vi "stitchingModeSimple_KJM.vi"(9 "Data In":dbl[][][](array[numeric])) -> (2 "Stitched Data Out":dbl[][](array[numeric]))   [LabVIEW 2020]
doc: "Stitches spectra based on simple cut-off modus."
uses:
  CCD.lvclass/CCD.ctl
  4c98e68f-fed8-44bd-a6f6-c5aabdf5d44d.vi
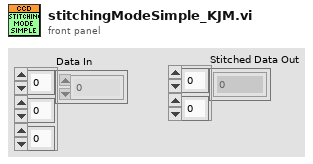
[diagram p1: front panel]
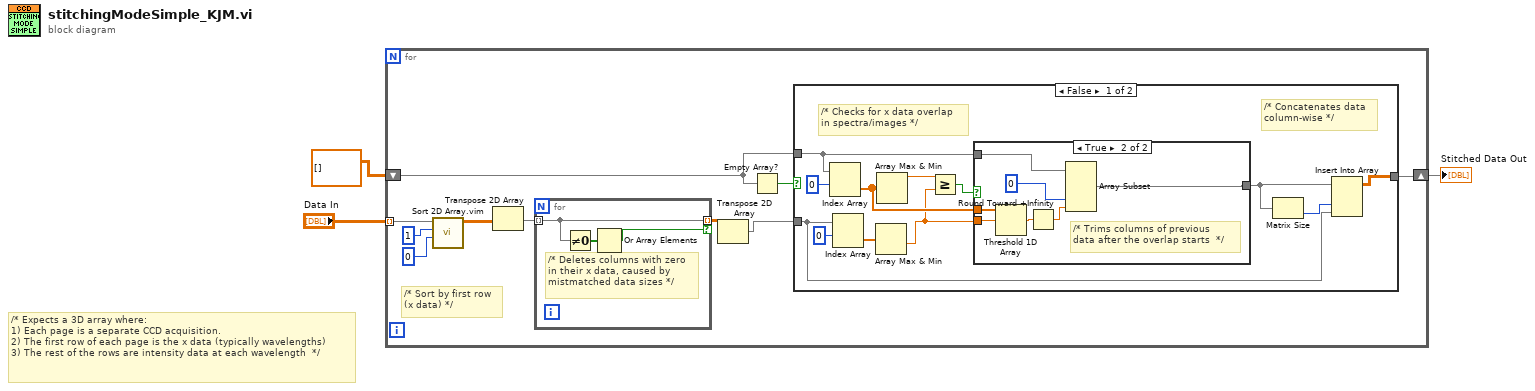
[diagram p0: block diagram]
diagram:
  # "/* Expects a 3D array where:\n1) Each page is a separate CCD acquisition.\n2) The first row of each page is the x data (typically wavelengths)\n3) The rest of the rows are intensity data at each wavelength  */"
  n1 = for {
    tunnel: "Data In" -> [w6] mode=indexing
    shift-right: [w13] -> w2
    shift-left: dbl[][] [] ("Empty Array") -> [w11]
    # "/* Sort by first row \n(x data) */"
    n2 = call "Sort 2D Array.vim"("index"=0, "dimension to index (column)"=1 ("index"), "2D array"=w6) -> ("sorted 2D array"=w5:dbl[][])  [unwired: 7 in, 1 out]
    n3 = Transpose 2D Array(2D array=w5) -> (transposed array=w10:dbl[][])
    n4 = for {
      tunnel: w10 -> [w15] mode=indexing
      tunnel: [w15] -> w9 mode=indexing if=w16
      # "/* Deletes columns with zero\nin their x data, caused by\nmistmatched data sizes */"
      n5 = Not Equal To 0?(x=w15) -> (x != 0?=w14:bool[])
      n6 = Or Array Elements(Boolean array=w14) -> (logical OR=w16:bool)
    }
    n7 = Transpose 2D Array(2D array=w9) -> (transposed array=w4:dbl[][])
    n8 = Empty Array?(array=w11) -> (empty?=w12:bool)
    n9 = case shown="False" w12 {
      tunnel: [w17 w37] -> w13
      tunnel: w4 -> [w25 w37]
      tunnel: w11 -> [w23 _]
      frame False {
        # "/* Concatenates data \ncolumn-wise */"
        # "/* Checks for x data overlap \nin spectra/images */"
        n10 = Index Array(array=w23, index (row)=0) -> (element=w22:dbl[])  [unwired: 1 in]
        n11 = Index Array(array=w25, index (row)=0) -> (element=w26:dbl[])  [unwired: 1 in]
        n12 = Array Max & Min(array=w26) -> (min value=w20:dbl)  [unwired: 3 out]
        n13 = Array Max & Min(array=w22) -> (max value=w21:dbl)  [unwired: 3 out]
        n14 = Greater Or Equal?(x=w21, y=w20) -> (x >= y?=w19:bool)
        n15 = case shown="True" w19 {
          tunnel: w23 -> [w29 w34]
          tunnel: [w29 w33] -> w18
          tunnel: w20 -> [_ w32]
          tunnel: w22 -> [_ w31]
          frame False {
            # "/* Passes previous data if \nthere is no overlap */"
          }
          frame True {
            # "/* Trims columns of previous \ndata after the overlap starts  */"
            n16 = Threshold 1D Array(2:w32, 3:w31) -> (0:w30:dbl)  [unwired: 1 in]
            n17 = Round Toward +Infinity(x=w30) -> (ceil(x): smallest int >= x=w35:dbl)
            n18 = Array Subset(array=w34, index (col)=0 ("index"), length (col)=w35) -> (w33:dbl[][])  [unwired: 2 in]
          }
        }
        n19 = Matrix Size(0:w18) -> (2:w24:i32)  [unwired: 1 out]
        n20 = Insert Into Array(array=w18, index (col)=w24, new element=w25) -> (w17:dbl[][])  [unwired: 1 in]
      }
      frame True {
        # "/* This case will run on the first loop iteration */"
      }
    }
  }
  "Stitched Data Out" <- w2
